vi "SwerveWheelHeadingCalc.vi"(9 "DriveIn":dbl, 10 "Target":dbl, 11 "Current":dbl) -> (2 "DriveOut":dbl, 3 "TargetFinal":dbl)   [LabVIEW 2017]
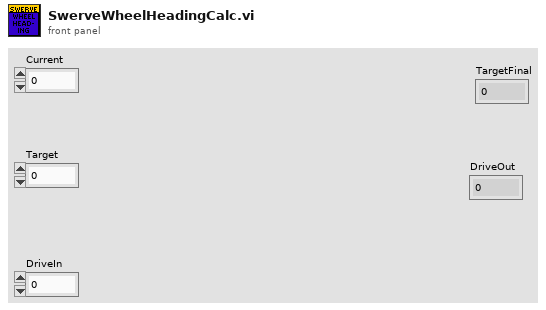
[diagram p1: front panel]
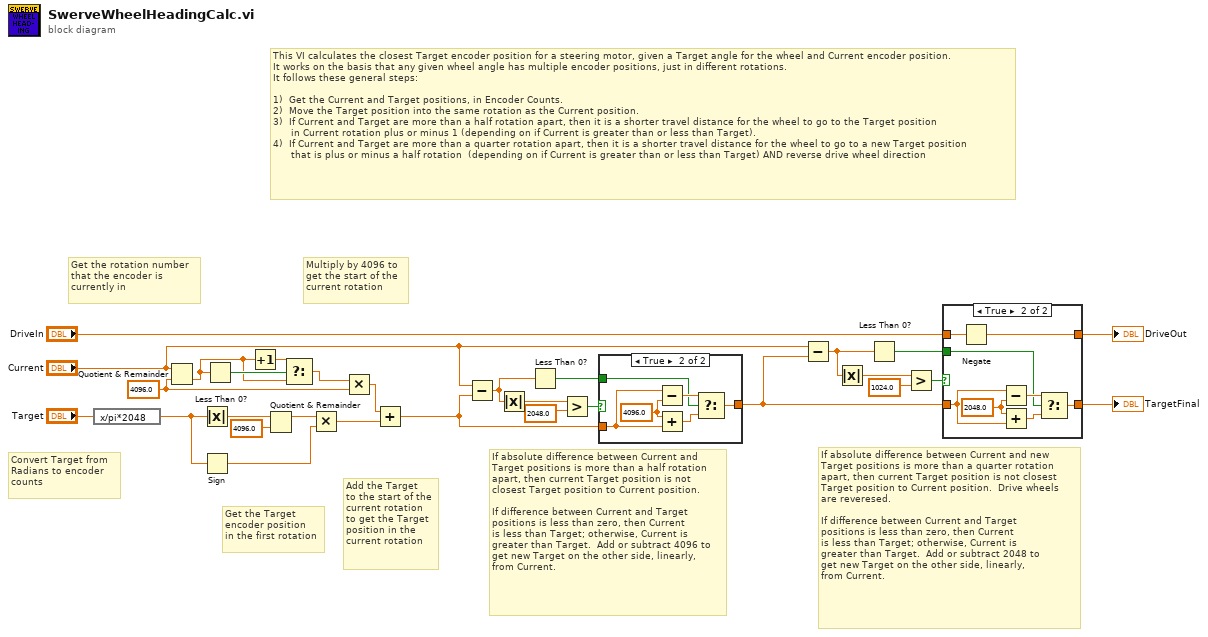
[diagram p0: block diagram]
diagram:
  w27 = 4096.0 ("y")
  # "This VI calculates the closest Target encoder position for a steering motor, given a Target angle for the wheel and Current encoder position.\nIt works on the basis that any given wheel angle has multiple encoder positions, just in different rotations.\nIt follows these general steps:\n\n1)  Get the Current and Target positions, in Encoder Counts.\n2)  Move the Target position into the same rotation as the Current position.\n3)  If Current and Target are more than a half rotation apart, then it is a shorter travel distance for the wheel to go to the Target position\n      in Current rotation plus or minus 1 (depending on if Current is greater than or less than Target).\n4)  If Current and Target are more than a quarter rotation apart, then it is a shorter travel distance for the wheel to go to a new Target position\n      that is plus or minus a half rotation  (depending on if Current is greater than or less than Target) AND reverse drive wheel direction"
  # "If absolute difference between Current and new\nTarget positions is more than a quarter rotation\napart, then current Target position is not closest\nTarget position to Current position.  Drive wheels\nare reveresed.\n\nIf difference between Current and Target\npositions is less than zero, then Current\nis less than Target; otherwise, Current is\ngreater than Target.  Add or subtract 2048 to\nget new Target on the other side, linearly,\nfrom Current."
  # "If absolute difference between Current and\nTarget positions is more than a half rotation\napart, then current Target position is not\nclosest Target position to Current position.\n\nIf difference between Current and Target\npositions is less than zero, then Current\nis less than Target; otherwise, Current is\ngreater than Target.  Add or subtract 4096 to\nget new Target on the other side, linearly,\nfrom Current."
  # "Multiply by 4096 to\nget the start of the\ncurrent rotation"
  # "Add the Target\nto the start of the\ncurrent rotation\nto get the Target\nposition in the\ncurrent rotation"
  # "Get the Target\nencoder position\nin the first rotation"
  # "Get the rotation number\nthat the encoder is\ncurrently in"
  # "Convert Target from\nRadians to encoder\ncounts"
  n1 = expression code="x/pi*2048"("Target") -> (w4:dbl)
  n2 = Quotient & Remainder(x="Current", y=w27) -> (floor(x/y)=w7:dbl)  [unwired: 1 out]
  n3 = Absolute Value(x=w4) -> (abs(x)=w5:dbl)
  n4 = Sign(1:w4) -> (0:w3:dbl)
  n5 = Less Than 0?(x=w7) -> (x < 0?=w8:bool)
  n6 = Increment(x=w7) -> (x+1=w9:dbl)
  n7 = Quotient & Remainder(x=w5, y=4096.0) -> (x-y*floor(x/y)=w2:dbl)  [unwired: 1 out]
  n8 = Select(t=w9, s=w8, f=w7) -> (s? t:f=w6:dbl)
  n9 = Multiply(x=w2, y=w3) -> (x*y=w1:dbl)
  n10 = Multiply(x=w6, y=w27) -> (x*y=w26:dbl)
  n11 = Add(x=w26, y=w1) -> (x+y=w21:dbl)
  n12 = Subtract(x="Current", y=w21) -> (x-y=w25:dbl)
  n13 = Absolute Value(x=w25) -> (abs(x)=w24:dbl)
  n14 = Less Than 0?(x=w25) -> (x < 0?=w20:bool)
  n15 = Greater?(x=w24, y=2048.0) -> (0:w22:bool)
  n16 = case shown="True" w22 {
    tunnel: w21 -> [w30 w35]
    tunnel: w20 -> [_ w32]
    tunnel: [w30 w31] -> w13
    frame False {
    }
    frame True {
      w36 = 4096.0 ("y")
      n17 = Subtract(x=w35, y=w36) -> (x-y=w34:dbl)
      n18 = Add(x=w36, y=w35) -> (x+y=w33:dbl)
      n19 = Select(t=w34, s=w32, f=w33) -> (s? t:f=w31:dbl)
    }
  }
  n20 = Subtract(x="Current", y=w13) -> (x-y=w19:dbl)
  n21 = Absolute Value(x=w19) -> (abs(x)=w17:dbl)
  n22 = Less Than 0?(x=w19) -> (x < 0?=w15:bool)
  n23 = Greater?(x=w17, y=1024.0) -> (0:w16:bool)
  n24 = case shown="True" w16 {
    tunnel: w15 -> [_ w39]
    tunnel: "DriveIn" -> [w37 w46]
    tunnel: [w37 w45] -> w14
    tunnel: w13 -> [w38 w41]
    tunnel: [w38 w40] -> w12
    frame False {
    }
    frame True {
      w42 = 2048.0 ("x")
      n25 = Negate(x=w46) -> (-x=w45:dbl)
      n26 = Subtract(x=w41, y=w42) -> (x-y=w44:dbl)
      n27 = Add(x=w42, y=w41) -> (x+y=w43:dbl)
      n28 = Select(t=w44, s=w39, f=w43) -> (s? t:f=w40:dbl)
    }
  }
  "TargetFinal" <- w12
  "DriveOut" <- w14
